vi "create.vi"(8 "error in (no error)":errorcluster, 11 "Summary":refnum<vi>) -> (0 "error out":errorcluster, 3 "GoalUserInterface out":refnum<class "SingleSelectMCLBAdapter.lvclass">)   [LabVIEW 2020, in "SingleSelectMCLBAdapter.lvclass"]
uses:
  SingleSelectMCLBAdapter.lvclass
  C:/GitRepos/Filthy-Lucre-Budgetizer/source/support/classes/AbstractMultiColumnListBoxAdapter/AbstractMultiColumnListBoxAdapter.lvclass
  SingleSelectMCLBAdapter.lvclass/SingleSelectMCLBAdapter.ctl
  AbstractMultiColumnListBoxAdapter/AbstractMultiColumnListBoxAdapter.lvclass
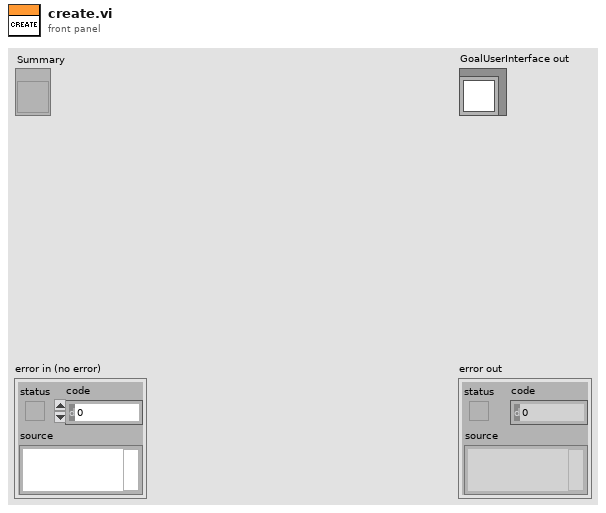
[diagram p1: front panel]
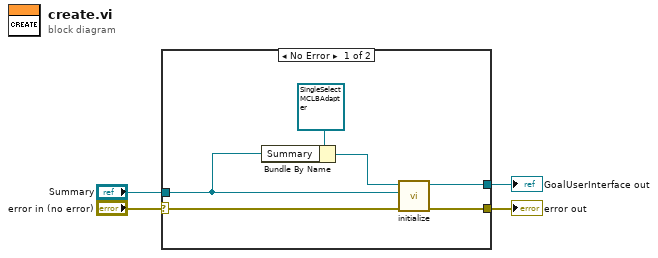
[diagram p0: block diagram]
diagram:
  n1 = case shown="No Error" "error in (no error)" {
    selector: "error in (no error)" -> [w6 w11]
    tunnel: [w5 w11] -> w3
    tunnel: [w8 _] -> w2
    tunnel: "Summary" -> [w7 _]
    frame No Error {
      n2 = Bundle By Name(cluster=refnum<class "SingleSelectMCLBAdapter.lvclass"> refnum ("GoalUserInterface in"), "Summary"=w7) -> (w9:refnum<class "SingleSelectMCLBAdapter.lvclass">)
      n3 = call "initialize.vi"("error in (no error)"=w6, "MCListbox Refnum"=w7, "AbstractMultiColumnListBoxAdapter in"=w9) -> ("error out"=w5:errorcluster, "AbstractMultiColumnListBoxAdapter out"=w8:refnum<class "SingleSelectMCLBAdapter.lvclass">)  [unwired: 7 in]
    }
    frame Error {
    }
  }
  "error out" <- w3
  "GoalUserInterface out" <- w2
